vi "Winch.vi"(6 "ElevatorButtonDown":i32=4, 7 "elevator height":dbl, 8 "WinchButton":i32=3, 9 "ElevatorButtonUp":i32=2, 10 "WinchSpeed":dbl=0.4, 11 "ElevatorSpeed":dbl=0.3) -> ()   [LabVIEW 2019]
uses:
  <vilib>/Rock Robotics/WPI/Solenoid/WPI_SolenoidValue.ctl
  <vilib>/Rock Robotics/WPI/Utilities/WPI_GetSetVariantRefNum.vi
  <vilib>/Rock Robotics/WPI/Solenoid/WPI_SolenoidSetEnum.vi
  <vilib>/Rock Robotics/Network Tables/NT Read Boolean.vi
panel:
  in  "elevator height 2":dbl
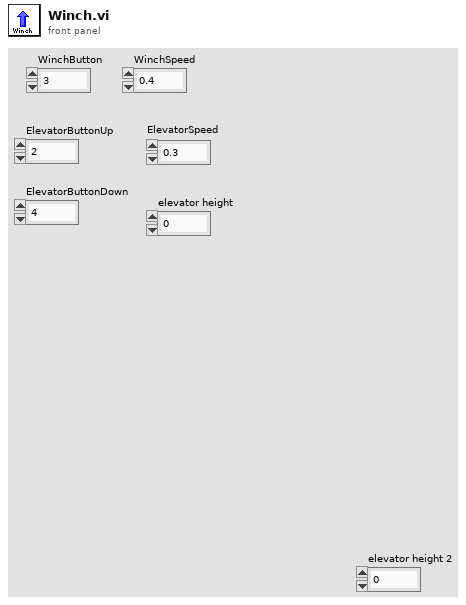
[diagram p1: front panel]
types:
  T1 = typedef "WPI_MotorControlDeviceRef.ctl" = cluster{"DeviceStatus":errorcluster, "Type":T2, "PWM":cluster{"PWM Channel":T3, "DeadBand":T4}, "CAN":cluster{"Device Number":u8, "SetOutput VI Ref":variant, "GetOutput VI Ref":variant, "Enable VI Ref":variant, "Disable VI Ref":variant, "Data":variant}, "Invert":bool, "DIO PWM":cluster{"PWM \"Enable\" Channel":T3, "DIOChannel":T5, "PWM Rate":dbl}}
  T2 = typedef "WPI_MotorControlType.ctl" = enum16{"PWM", "CAN", "DIO PWM"}
  T3 = typedef "FPGA_DIOPWMChannel.ctl" = enum8{"PWM 0", "PWM 1", "PWM 2", "PWM 3", "PWM 4", "PWM 5", "PWM 6", "PWM 7", "PWM 8", "PWM 9", "PWM MXP 0", "PWM MXP 1", "PWM MXP 2", "PWM MXP 3", "PWM MXP 4", "PWM MXP 5", "PWM MXP 6", "PWM MXP 7", "PWM MXP 8", "PWM MXP 9", "Invalid"}
  T4 = typedef "WPI_PWMDeadband.ctl" = cluster{"Name":string, "maxPositivePwm":i32, "minPositivePwm":i32, "centerPwm":i32, "maxNegativePwm":i32, "minNegativePwm":i32, "angularRange":u16}
  T5 = typedef "FPGA_DIOChannel.ctl" = enum8{"DIO 0", "DIO 1", "DIO 2", "DIO 3", "DIO 4", "DIO 5", "DIO 6", "DIO 7", "DIO 8", "DIO 9", "DIO MXP 0", "DIO MXP 1", "DIO MXP 2", "DIO MXP 3", "DIO MXP 4", "DIO MXP 5", "DIO MXP 6", "DIO MXP 7", "DIO MXP 8", "DIO MXP 9", "DIO MXP 10", "DIO MXP 11", "DIO MXP 12", "DIO MXP 13", "DIO MXP 14", "DIO MXP 15", "SPI Port CS1", "SPI Port CS2", "SPI Port CS3", "SPI Port MISO", "SPI Port MOSI", "Invalid"}
  T6 = typedef "WPI_JoystickDevRef.ctl" = cluster{"Device":T7}
  T7 = typedef "WPI_JoystickDeviceEnum.ctl" = enum16{"USB 0", "USB 1", "USB 2", "USB 3", "USB 4", "USB 5"}
  T8 = typedef "WPI_SolenoidValue.ctl" = enum16{"Off", "On", "Forward", "Reverse"}
  T9 = typedef "WPI_SolenoidDevRef.ctl" = cluster{"DevStatus":errorcluster, "Pneumatics Control Module":u8, "Forward Solenoid Channel":T10, "Reverse Solenoid Channel":T10}
  T10 = typedef "WPI_SolenoidChannel.ctl" = enum8{"Solenoid 0", "Solenoid 1", "Solenoid 2", "Solenoid 3", "Solenoid 4", "Solenoid 5", "Solenoid 6", "Solenoid 7", "Invalid"}
  T11 = typedef "WPI_EncoderDevRef.ctl" = cluster{"DevStatus":errorcluster, "EncoderIndex":T12, "CounterIndex":T13, "DistancePerCount":dbl, "Decoding Type":T14}
  T12 = typedef "FPGA_EncoderIdx.ctl" = enum8{"Enc 0", "Enc 1", "Enc 2", "Enc 3", "Enc 4", "Enc 5", "Enc 6", "Enc 7", "Invalid"}
  T13 = typedef "FPGA_CounterCtrSystemIndex.ctl" = enum8{"Ctr 0", "Ctr 1", "Ctr 2", "Ctr 3", "Ctr 4", "Ctr 5", "Ctr 6", "Ctr 7", "Invalid"}
  T14 = typedef "WPI_EncoderType.ctl" = enum16{"1x", "2x", "4x"}
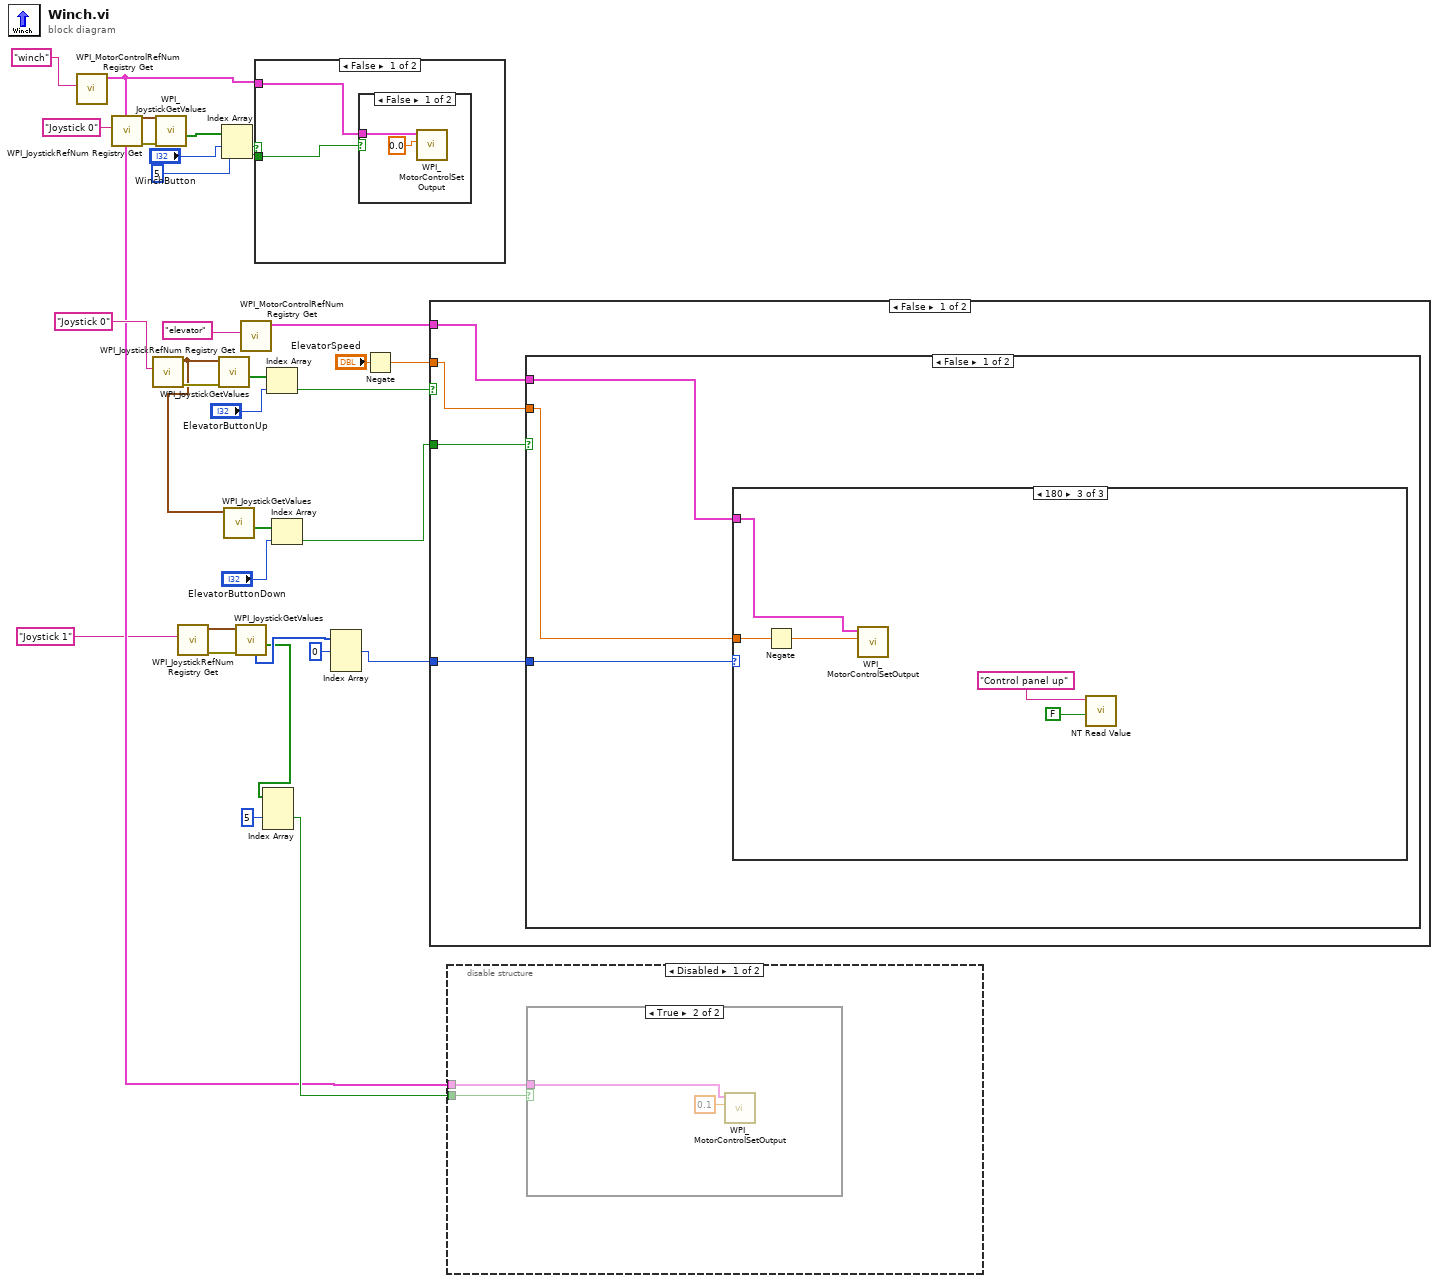
[diagram p0: block diagram]
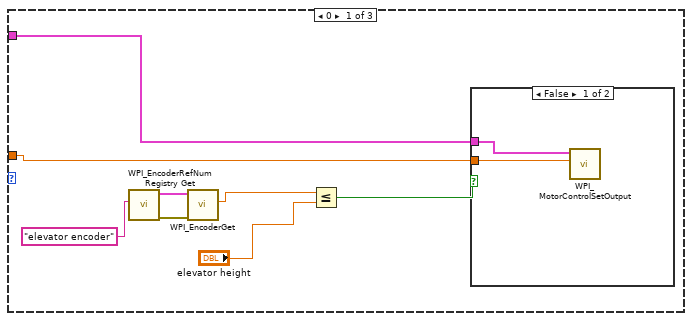
[diagram p4: hidden frame]
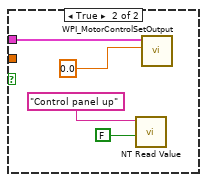
[diagram p5: hidden frame]
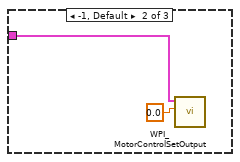
[diagram p6: hidden frame]
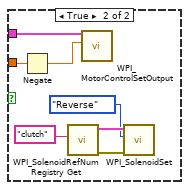
[diagram p7: hidden frame]
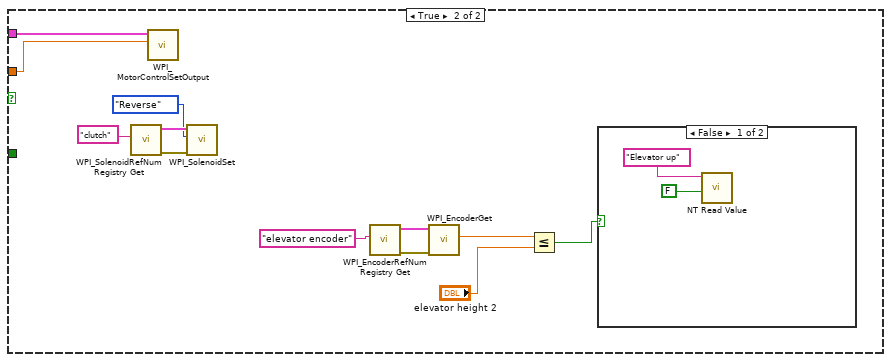
[diagram p8: hidden frame]
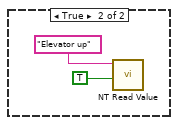
[diagram p9: hidden frame]
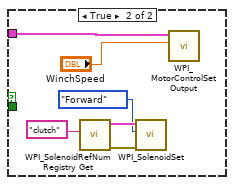
[diagram p11: hidden frame]
diagram:
  n1 = call <vilib>:"WPI_MotorControlRefNum Registry Get.vi"("refnum name"="winch") -> ("MotorControlDevRef"=w8:T1)  [unwired: 9 in, 1 out]
  n2 = call <vilib>:"WPI_JoystickRefNum Registry Get.vi"("refnum name"="Joystick 0") -> ("error out"=w31:errorcluster, "JoystickDevRef"=w30:T6)  [unwired: 9 in]
  n3 = call <vilib>:"WPI_JoystickRefNum Registry Get.vi"("refnum name"="Joystick 0") -> ("error out"=w26:errorcluster, "JoystickDevRef"=w5:T6)  [unwired: 9 in]
  n4 = call <vilib>:"WPI_JoystickGetValues.vi"("error in (no error)"=w31, "JoystickDevRef"=w30) -> ("Buttons"=w29:bool[])  [unwired: 5 in, 4 out]
  n5 = call <vilib>:"WPI_JoystickRefNum Registry Get.vi"("refnum name"="Joystick 1") -> ("error out"=w4:errorcluster, "JoystickDevRef"=w3:T6)  [unwired: 9 in]
  n6 = call <vilib>:"WPI_JoystickGetValues.vi"("error in (no error)"=w26, "JoystickDevRef"=w5) -> ("Buttons"=w25:bool[])  [unwired: 5 in, 4 out]
  n7 = Index Array(array=w29, index #1="WinchButton", index #2=5 ("index")) -> (element #1=w28:bool, element #2=w6:bool)
  n8 = call <vilib>:"WPI_JoystickGetValues.vi"("JoystickDevRef"=w5) -> ("Buttons"=w20:bool[])  [unwired: 6 in, 4 out]
  n9 = call <vilib>:"WPI_JoystickGetValues.vi"("error in (no error)"=w4, "JoystickDevRef"=w3) -> ("Buttons"=w11:bool[], "POVs"=w16:i16[])  [unwired: 5 in, 3 out]
  n10 = call <vilib>:"WPI_MotorControlRefNum Registry Get.vi"("refnum name"="elevator") -> ("MotorControlDevRef"=w23:T1)  [unwired: 9 in, 1 out]
  n11 = case shown="False" w28 {
    tunnel: w8 -> [w34 w41]
    tunnel: w6 -> [w33 _]
    frame False {
      n12 = case shown="False" w33 {
        tunnel: w34 -> [w35 _]
        frame False {
          n13 = call <vilib>:"WPI_MotorControlSetOutput.vi"("Output"=0.0, "MotorControlDevRef"=w35) -> ()  [unwired: 7 in, 3 out]
        }
        frame True {
        }
      }
    }
    frame True {
      n14 = call <vilib>:"WPI_SolenoidRefNum Registry Get.vi"("refnum name"="clutch") -> ("error out"=w39:errorcluster, "SolenoidDevRef"=w38:T9)  [unwired: 9 in]
      n15 = call-poly <vilib>:"WPI_SolenoidSet.vi"("error in (no error)"=w39, "Value"=WPI_SolenoidValue."Forward", "SolenoidDevRef"=w38) -> ()  [unwired: 7 in, 2 out]
      n16 = call <vilib>:"WPI_MotorControlSetOutput.vi"("Output"="WinchSpeed", "MotorControlDevRef"=w41) -> ()  [unwired: 7 in, 3 out]
    }
  }
  n17 = Index Array(array=w11, index #2=5 ("index")) -> (element #2=w9:bool)  [unwired: 2 in, 2 out]
  n18 = Index Array(array=w25, index="ElevatorButtonUp") -> (element=w24:bool)
  n19 = Index Array(array=w20, index="ElevatorButtonDown") -> (element=w18:bool)
  n20 = Index Array(array=w16, index #1=0 ("index")) -> (element #1=w14:i16)  [unwired: 2 in, 2 out]
  n21 = Negate(x="ElevatorSpeed") -> (-x=w1:dbl)
  n22 = case shown="False" w24 {
    tunnel: w23 -> [w43 w89]
    tunnel: w18 -> [w46 _]
    tunnel: w1 -> [w45 w84]
    tunnel: w14 -> [w44 _]
    frame False {
      n23 = case shown="False" w46 {
        tunnel: w43 -> [w48 w77]
        tunnel: w45 -> [w47 w72]
        tunnel: w44 -> [w49 _]
        frame False {
          n24 = case shown="180" w49 {
            tunnel: w48 -> [w57 w64 w70]
            tunnel: w47 -> [w50 _ w69]
            frame 0 {
              n25 = call <vilib>:"WPI_EncoderRefNum Registry Get.vi"("refnum name"="elevator encoder") -> ("error out"=w56:errorcluster, "EncoderDevRef"=w55:T11)  [unwired: 9 in]
              n26 = call <vilib>:"WPI_EncoderGet.vi"("error in (no error)"=w56, "EncoderDevRef"=w55) -> ("Distance"=w54:dbl)  [unwired: 4 in, 5 out]
              n27 = Less Or Equal?(x=w54, y="elevator height") -> (x <= y?=w53:bool)
              n28 = case shown="False" w53 {
                tunnel: w57 -> [w59 w62]
                tunnel: w50 -> [w58 _]
                frame False {
                  n29 = call <vilib>:"WPI_MotorControlSetOutput.vi"("Output"=w58, "MotorControlDevRef"=w59) -> ()  [unwired: 7 in, 3 out]
                }
                frame True {
                  n30 = call-poly <vilib>:"NT Read Value.vi"("Default Value"=FALSE, "Name"="Control panel up") -> ()  [unwired: 8 in, 2 out]
                  n31 = call <vilib>:"WPI_MotorControlSetOutput.vi"("Output"=0.0, "MotorControlDevRef"=w62) -> ()  [unwired: 7 in, 3 out]
                }
              }
            }
            frame -1, Default {
              n32 = call <vilib>:"WPI_MotorControlSetOutput.vi"("Output"=0.0, "MotorControlDevRef"=w64) -> ()  [unwired: 7 in, 3 out]
            }
            frame 180 {
              n33 = Negate(x=w69) -> (-x=w66:dbl)
              n34 = call <vilib>:"WPI_MotorControlSetOutput.vi"("Output"=w66, "MotorControlDevRef"=w70) -> ()  [unwired: 7 in, 3 out]
              n35 = call-poly <vilib>:"NT Read Value.vi"("Default Value"=FALSE, "Name"="Control panel up") -> ()  [unwired: 8 in, 2 out]
            }
          }
        }
        frame True {
          n36 = Negate(x=w72) -> (-x=w71:dbl)
          n37 = call <vilib>:"WPI_SolenoidRefNum Registry Get.vi"("refnum name"="clutch") -> ("error out"=w75:errorcluster, "SolenoidDevRef"=w74:T9)  [unwired: 9 in]
          n38 = call <vilib>:"WPI_MotorControlSetOutput.vi"("Output"=w71, "MotorControlDevRef"=w77) -> ()  [unwired: 7 in, 3 out]
          n39 = call-poly <vilib>:"WPI_SolenoidSet.vi"("error in (no error)"=w75, "Value"=WPI_SolenoidValue."Reverse", "SolenoidDevRef"=w74) -> ()  [unwired: 7 in, 2 out]
        }
      }
    }
    frame True {
      n40 = call <vilib>:"WPI_SolenoidRefNum Registry Get.vi"("refnum name"="clutch") -> ("error out"=w87:errorcluster, "SolenoidDevRef"=w86:T9)  [unwired: 9 in]
      n41 = call <vilib>:"WPI_MotorControlSetOutput.vi"("Output"=w84, "MotorControlDevRef"=w89) -> ()  [unwired: 7 in, 3 out]
      n42 = call-poly <vilib>:"WPI_SolenoidSet.vi"("error in (no error)"=w87, "Value"=WPI_SolenoidValue."Reverse", "SolenoidDevRef"=w86) -> ()  [unwired: 7 in, 2 out]
      n43 = call <vilib>:"WPI_EncoderRefNum Registry Get.vi"("refnum name"="elevator encoder") -> ("error out"=w83:errorcluster, "EncoderDevRef"=w82:T11)  [unwired: 9 in]
      n44 = call <vilib>:"WPI_EncoderGet.vi"("error in (no error)"=w83, "EncoderDevRef"=w82) -> ("Distance"=w80:dbl)  [unwired: 4 in, 5 out]
      n45 = Less Or Equal?(x=w80, y="elevator height 2") -> (x <= y?=w78:bool)
      n46 = case shown="False" w78 {
        frame False {
          n47 = call-poly <vilib>:"NT Read Value.vi"("Default Value"=FALSE, "Name"="Elevator up") -> ()  [unwired: 8 in, 2 out]
        }
        frame True {
          n48 = call-poly <vilib>:"NT Read Value.vi"("Default Value"=TRUE, "Name"="Elevator up") -> ()  [unwired: 8 in, 2 out]
        }
      }
    }
  }
  n49 = disable-structure shown="Disabled" {
    disable-tunnel: w9 -> [w95 _]
    disable-tunnel: w8 -> [w94 _]
    frame Disabled {
      n50 = case shown="True" w95 {
        tunnel: w94 -> [_ w97]
        frame False {
        }
        frame True {
          n51 = call <vilib>:"WPI_MotorControlSetOutput.vi"("Output"=0.1, "MotorControlDevRef"=w97) -> ()  [unwired: 7 in, 3 out]
        }
      }
    }
    frame Enabled {
    }
  }
